vi "AIDI-Create Tasks (AI).vi"(0 "Channels":string[](array[string]), 11 "error in (no error)":errorcluster) -> (4 "Task Specs":T1[](array[typedef]), 15 "error out":errorcluster)   [LabVIEW 2020]
doc: "Creates (at most) one AO and one AI task per board. Loops through channels and decodes device and \"direction\" (i.e. AO or AI) for each channel. Creates a new task if device and direction have not been used. Otherwise, adds current channel to existing task."
uses:
  Typedefs/AIDI-Task Specification.ctl
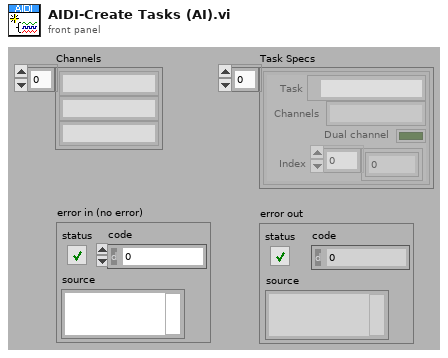
[diagram p1: front panel]
types:
  T1 = typedef "AIDI-Task Specification.ctl" = cluster{"Task":refnum<k21>, "Channels":string, "Dual channel":bool, "Index":i32[]}
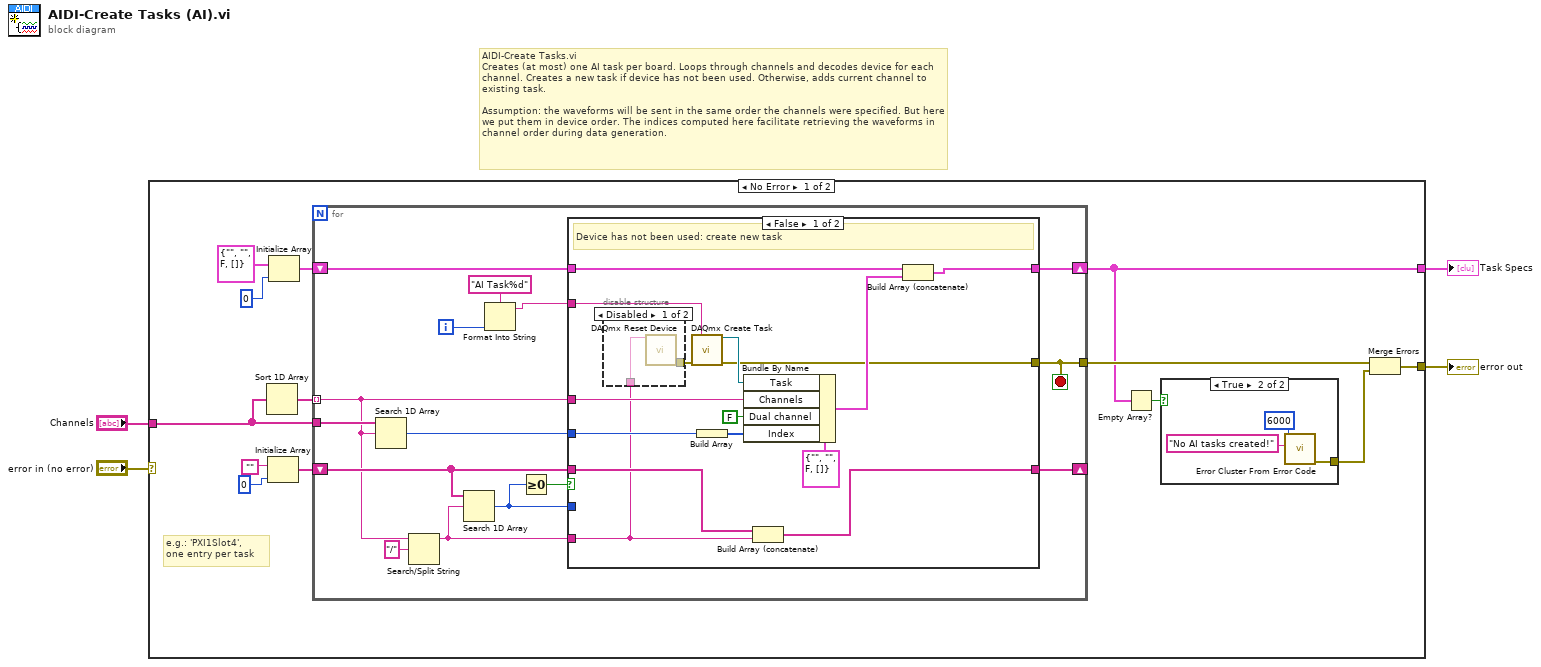
[diagram p0: block diagram]
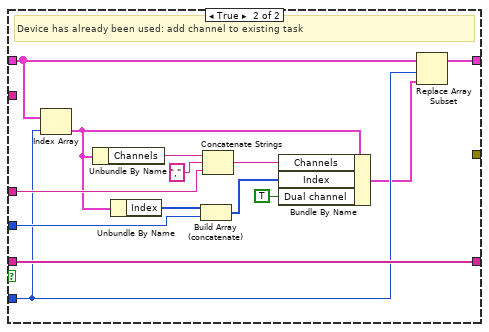
[diagram p3: hidden frame]
diagram:
  # "AIDI-Create Tasks.vi\nCreates (at most) one AI task per board. Loops through channels and decodes device for each channel. Creates a new task if device has not been used. Otherwise, adds current channel to existing task.\n\nAssumption: the waveforms will be sent in the same order the channels were specified. But here we put them in device order. The indices computed here facilitate retrieving the waveforms in channel order during data generation."
  n1 = case shown="No Error" "error in (no error)" {
    selector: "error in (no error)" -> [_ w67]
    tunnel: "Channels" -> [w15 _]
    tunnel: [w6 w67] -> w4
    tunnel: [w5 _] -> w2
    frame No Error {
      # "e.g.: 'PXI1Slot4',\none entry per task"
      n2 = Sort 1D Array(array=w15) -> (sorted array=w16:string[])
      n3 = Initialize Array("", 0 ("dimension size")) -> (w10:string[])
      n4 = Initialize Array(T1 {"Task"="", "Channels"="", "Dual channel"=FALSE, "Index"=[]} ("Task Specification"), 0) -> (w12:T1[])
      n5 = for {
        tunnel: w16 -> [w26] mode=indexing
        shift-right: [w28] -> _
        shift-left: w10 -> [w30]
        tunnel: w15 -> [w27]
        shift-right: [w23] -> w5
        shift-left: w12 -> [w24]
        tunnel: [w22] -> w8
        i -> [w19]
        stop <- w22 stop-if-true
        n6 = Search 1D Array(1D array=w27, element=w26) -> (index of element=w25:i32)  [unwired: 1 in]
        n7 = Search/Split String(string=w26, search string/char (-)="/") -> (substring before match=w21:string)  [unwired: 1 in, 2 out]
        n8 = Search 1D Array(1D array=w30, element=w21) -> (index of element=w29:i32)  [unwired: 1 in]
        n9 = Format Into String(format string="AI Task%d", w19) -> (resulting string=w18:string)  [unwired: 2 in, 1 out]
        n10 = Greater Or Equal To 0?(x=w29) -> (x >= 0?=w31:bool)
        n11 = case shown="False" w31 {
          tunnel: w30 -> [w47 w63]
          tunnel: w21 -> [w34 _]
          tunnel: w26 -> [w43 w60]
          tunnel: w29 -> [_ w51]
          tunnel: [w46 w63] -> w28
          tunnel: w25 -> [w41 w58]
          tunnel: w24 -> [w39 w53]
          tunnel: [w38 w52] -> w23
          tunnel: [w36 _] -> w22
          tunnel: w18 -> [w33 _]
          frame False {
            # "Device has not been used: create new task"
            n12 = disable-structure shown="Disabled" {
              disable-tunnel: [w49 _] -> w35
              disable-tunnel: w34 -> [w48 _]
              frame Disabled {
                n13 = call <vilib>:"DAQmx Reset Device.vi"("device in"=w48) -> ("error out"=w49:errorcluster)  [unwired: 14 in]
              }
              frame Enabled {
              }
            }
            n14 = call <vilib>:"DAQmx Create Task.vi"("new task name"=w33, "error in"=w35) -> ("task out"=w44:refnum<k21>, "error out"=w36:errorcluster)  [unwired: 12 in]
            n15 = Build Array(w41) -> (w40:i32[])
            n16 = Bundle By Name(cluster=T1 {"Task"="", "Channels"="", "Dual channel"=FALSE, "Index"=[]} ("Task Specification"), "Task"=w44, "Channels"=w43, "Dual channel"=FALSE, "Index"=w40) -> (w37:T1)
            n17 = Build Array (concatenate)(w47, w34) -> (w46:string[])
            n18 = Build Array (concatenate)(w39, w37) -> (w38:T1[])
          }
          frame True {
            # "Device has already been used: add channel to existing task"
            n19 = Index Array(array=w53, index=w51) -> (element=w57:T1)
            n20 = Unbundle By Name(w57) -> ("Channels"=w62:string)
            n21 = Unbundle By Name(w57) -> ("Index"=w59:i32[])
            n22 = Build Array (concatenate)(w59, w58) -> (w55:i32[])
            n23 = Concatenate Strings(w62, ",", w60) -> (w56:string)
            n24 = Bundle By Name(cluster=w57, "Channels"=w56, "Index"=w55, "Dual channel"=TRUE) -> (w50:T1)
            n25 = Replace Array Subset(array=w53, new element=w50, index=w51) -> (w52:T1[])
          }
        }
      }
      n26 = Empty Array?(array=w5) -> (empty?=w17:bool)
      n27 = case shown="True" w17 {
        tunnel: [_ w64] -> w7
        frame False {
        }
        frame True {
          n28 = call <vilib>:"Error Cluster From Error Code.vi"("error message (\"\")"="No AI tasks created!" ("error message (\"\")"), "error code (0)"=6000) -> ("error out"=w64:errorcluster)  [unwired: 7 in]
        }
      }
      n29 = Merge Errors(w8, w7) -> (w6:errorcluster)
    }
    frame Error {
    }
  }
  "error out" <- w4
  "Task Specs" <- w2
